vi "KlingerV2 ControlLimit.vi"(0 "Axe":u8(ring) items=["W", "X", "Y", "Z"], 1 "UnitDem":u8(ring) caption="Unités\nDemandées" items=["Pas", "mm", "ps", "Degré (°)"], 3 "error in":errorcluster) -> (5 "DataRange":T1 {"Increment" format="%#_1g"; "Maximum" format="%#_10g"; "Minimum" format="%#_10g"}, 6 "FormtPrec":cluster{"Format":u8, "Precision":u8} caption="Format &\nPrécision", 7 "error out":errorcluster)   [LabVIEW 2012]
doc: "Ce VI retourne la plage des données acceptable par le contrôleur en fonction de l'axe et de l'unité choisi. Il retourne le maximum, le minimum, l'incrément (résolution), et la précision d'affichage à appliquer au contrôle de consigne de déplacement, pour l'axe et l'unité en vigueur. Cela empêche la saisi de consigne hors limite."
uses:
  <userlib>/KlingerV2/KlingerV2 Params.ctl
  <userlib>/KlingerV2/KlingerV2 ConvUnitArr.vi
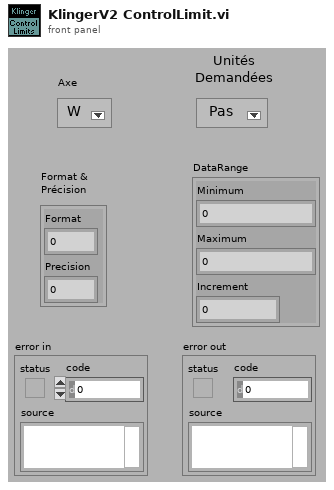
[diagram p1: front panel]
types:
  T1 = cluster{"Minimum":dbl, "Maximum":dbl, "Increment":dbl}
  T2 = typedef "KlingerV2 Params.ctl" = enum16{"Type", "Origine", "Encodeur", "TypeMouv", "FactConv", "Nom", "CorrParams", "KlingCtrlPar", "Speed", "Acc", "Avance", "Tous"}
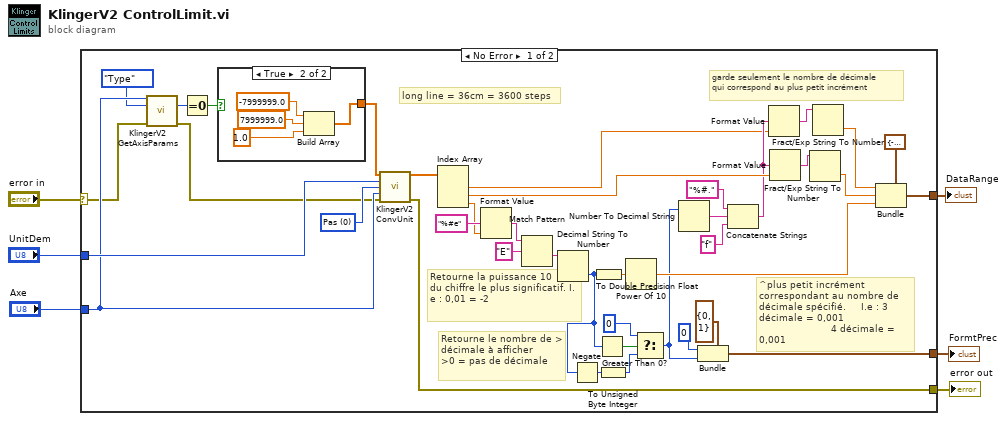
[diagram p0: block diagram]
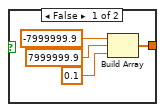
[diagram p2: hidden frame]
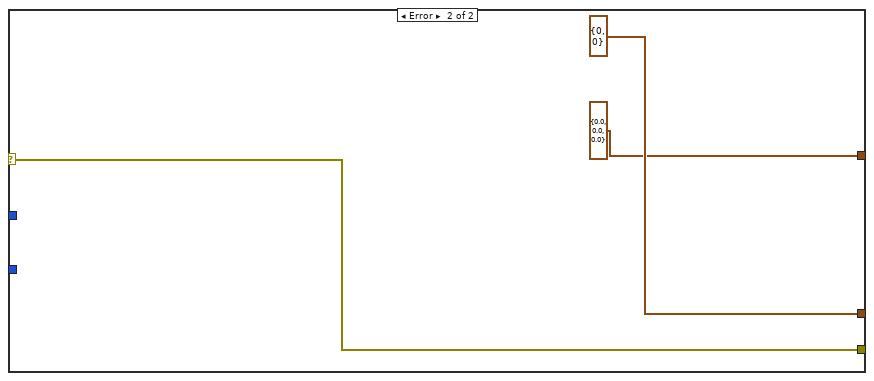
[diagram p3: hidden frame]
diagram:
  n1 = case shown="No Error" "error in" {
    selector: "error in" -> [w37 w56]
    tunnel: [w44 w56] -> w6
    tunnel: "Axe" -> [w41 _]
    tunnel: "UnitDem" -> [w43 _]
    tunnel: [w35 T1 {"Minimum"=0.0, "Maximum"=0.0, "Increment"=0.0} ("Data Range")] -> w2
    tunnel: [w32 cluster{"Format":u8, "Precision":u8} {"Format"=0, "Precision"=0} ("Format & Precision")] -> w1
    frame No Error {
      w42 = u8 0 items=["Pas", "mm", "ps", "Degré (°)"] ("UnitAct")
      # "long line = 36cm = 3600 steps"
      # "Retourne la puissance 10\ndu chiffre le plus significatif. I.e : 0,01 = -2"
      # "^plus petit incrément correspondant au nombre de décimale spécifié.     I.e : 3 décimale = 0,001\n                        4 décimale = 0,001"
      # "Retourne le nombre de > décimale à afficher\n>0 = pas de décimale"
      # "garde seulement le nombre de décimale\nqui correspond au plus petit incrément"
      n2 = call <userlib>:"KlingerV2 GetAxisParams.vi"("Axe"=w41, "Param"=KlingerV2_Params."Type", "error in"=w37) -> ("Type"=w40:i32, "error out"=w36:errorcluster)  [unwired: 3 in, 8 out]
      n3 = Equal To 0?(x=w40) -> (x = 0?=w39:bool)
      n4 = case shown="True" w39 {
        tunnel: [w46 w50] -> w38
        frame False {
          n5 = Build Array(-7999999.9 ("Minimum"), 7999999.9 ("Maximum"), 0.1 ("Increment")) -> (w46:dbl[])
        }
        frame True {
          n6 = Build Array(-7999999.0 ("Minimum"), 7999999.0 ("Minimum"), 1.0 ("Increment")) -> (w50:dbl[])
        }
      }
      n7 = call-poly <userlib>:"KlingerV2 ConvUnit.vi"("ParamAct"=w38, "UnitDem"=w43, "UnitAct"=w42, "Axe"=w41, "error in"=w36) -> ("ParamDem"=w31:dbl[], "error out"=w44:errorcluster)  [unwired: 9 in]
      n8 = Index Array(array=w31) -> (element #1=w19:dbl, element #2=w26:dbl, element #3=w27:dbl)  [unwired: 3 in]
      n9 = Format Value(format string="%#e", value (0)=w27) -> (output string=w28:string)  [unwired: 1 in]
      n10 = Match Pattern(string=w28, regular expression="E") -> (after substring=w15:string)  [unwired: 1 in, 3 out]
      n11 = Decimal String To Number(string=w15) -> (number=w9:i32)  [unwired: 2 in, 1 out]
      n12 = Negate(x=w9) -> (-x=w11:i32)
      n13 = To Double Precision Float(number=w9) -> (double precision float=w22:dbl)
      n14 = Greater Than 0?(x=w9) -> (x > 0?=w13:bool)
      n15 = To Unsigned Byte Integer(number=w11) -> (unsigned 8bit integer=w10:u8)
      n16 = Power Of 10(x=w22) -> (10^x=w14:dbl)
      n17 = Select(t=u8 0 ("Format"), s=w13, f=w10) -> (s? t:f=w8:u8)
      n18 = Number To Decimal String(number=w8) -> (decimal integer string=w21:string)  [unwired: 1 in]
      n19 = Bundle(cluster=cluster{"Format":u8, "Precision":u8} {"Format"=0, "Precision"=1} ("Format & Precision"), "Format"=u8 0, "Precision"=w8) -> (w32:cluster{"Format":u8, "Precision":u8})
      n20 = Concatenate Strings("%#." ("format string"), w21, "f" ("format string")) -> (w20:string)
      n21 = Format Value(format string=w20, value (0)=w19) -> (output string=w18:string)  [unwired: 1 in]
      n22 = Format Value(format string=w20, value (0)=w26) -> (output string=w17:string)  [unwired: 1 in]
      n23 = Fract/Exp String To Number(string=w17) -> (number=w25:dbl)  [unwired: 3 in, 1 out]
      n24 = Fract/Exp String To Number(string=w18) -> (number=w16:dbl)  [unwired: 3 in, 1 out]
      n25 = Bundle(cluster=T1 {"Minimum"=-7999999.9, "Maximum"=7999999.9, "Increment"=0.1} ("Data Range"), "Minimum"=w16, "Maximum"=w25, "Increment"=w14) -> (w35:T1)
    }
    frame Error {
    }
  }
  "error out" <- w6
  "DataRange" <- w2
  "FormtPrec" <- w1
